vi "WriteToRandomFile.vi"() -> ()   [LabVIEW 2026]
panel:
  out "Web Browser Control":string(html)
  out "text":string
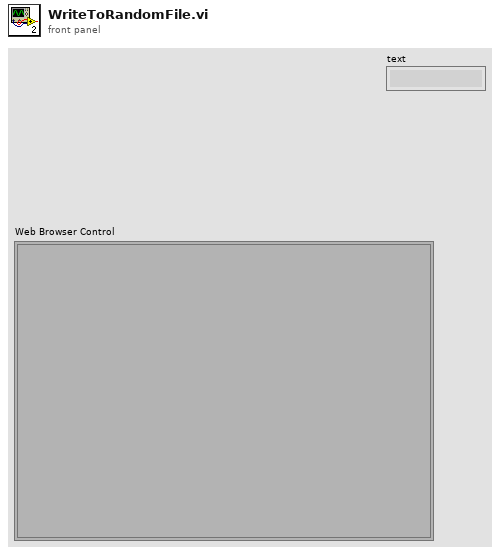
[diagram p1: front panel]
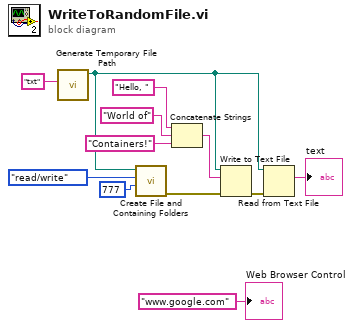
[diagram p0: block diagram]
diagram:
  n1 = call <vilib>:"Generate Temporary File Path.vi"("Temporary File Extension (tmp)"="txt") -> ("Unique Temporary File Path"=w2:path)  [unwired: 9 in, 1 out]
  n2 = call <vilib>:"Create File and Containing Folders.vi"("permissions"=i16 777, "access"=enum16{"read/write", "read-only", "write-only"}."read/write", "file path"=w2) -> ("error out"=w6:errorcluster)  [unwired: 7 in, 1 out]
  n3 = Concatenate Strings("Hello, " ("string"), "World of" ("string"), "Containers!" ("string")) -> (w5:string)
  n4 = Write to Text File(file (use dialog)=w2, text=w5, error in=w6) -> (error out=w3:errorcluster)  [unwired: 1 in, 2 out]
  n5 = Read from Text File(file (use dialog)=w2, error in=w3) -> (text=→"text":string)  [unwired: 2 in, 3 out]
  "Web Browser Control" <- "www.google.com" ("Web Browser Control")
